vi "1.2.3-ReadRequestSerial.vi"(10 "Sending":bool) -> ()   [LabVIEW 2010]
uses:
  <vilib>/eio/EIOMethodNode/EIOMethodNode.xnode
  <vilib>/rvi/eio/nirviEIOMethodImplementation/nirviEIOMethodImplementation.xnode
  <vilib>/rvi/eio/common/nirviEmuClasses.ctl
  1.0-Hindbrain Global.vi
  <vilib>/rvi/eio/common/nirviEmuTemplateMethod_noerrors.vi
panel:
  # "$VNRRG,08*7B,: 36 - 86 - 78 - 82 - 82 - 71 - 44 - 48 - 56 - 42 - 55 - 66"
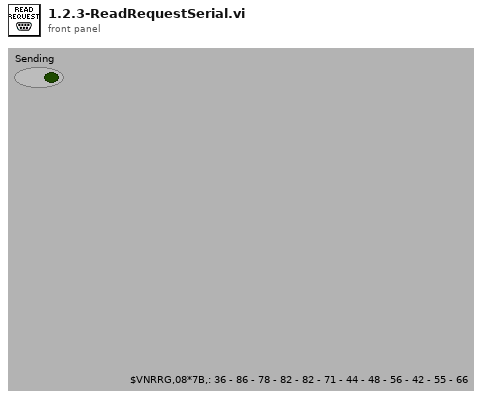
[diagram p1: front panel]
types:
  T1 = typedef "nirviEmuClasses.ctl" = enum16{"IO Read", "IO Write", "Method", "Property Read", "Property Write"}
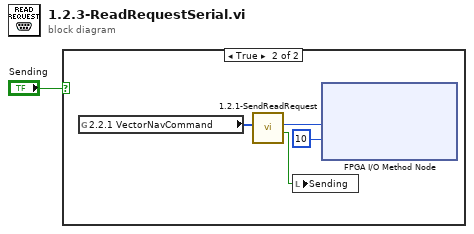
[diagram p0: block diagram]
diagram:
  n1 = case shown="True" "Sending" {
    frame False {
    }
    frame True {
      n2 = global read "1.0-Hindbrain Global.vi" "2.2.1 VectorNavCommand"() -> (w2:u8[])
      n3 = call "1.2.1-SendReadRequest.vi"("Command"=w2) -> ("Sending"=w3:bool, "Serial Byte"=w4:u8)  [unwired: 9 in]
      n4 = local write "Sending"(w3) -> ()
      n5 = xnode "FPGA I/O Method Node"("Data"=w4, "Timeout (ms)"=10) -> ()  [unwired: 1 in, 2 out]
    }
  }
